vi "Calc Panel Position.vi"(11 "窗格引用":refnum<vi>) -> (3 "Panel Position":T1)   [LabVIEW 2016]
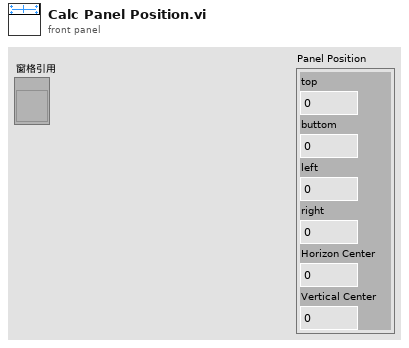
[diagram p1: front panel]
types:
  T1 = cluster{"top":i32, "buttom":i32, "left":i32, "right":i32, "Horizon Center":i32, "Vertical Center":i32}
  T2 = typedef "LVRectTypeDef.ctl" = cluster{"Left":i16, "Top":i16, "Right":i16, "Bottom":i16}
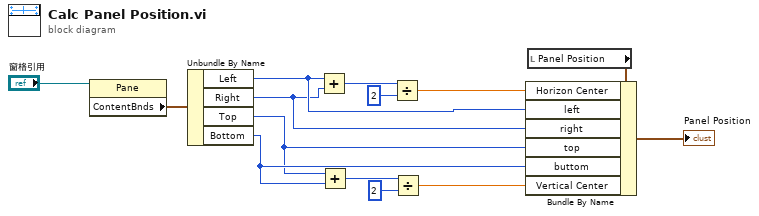
[diagram p0: block diagram]
diagram:
  n1 = property class="Pane"(reference="窗格引用") -> ("ContentBnds"=w10:T2)  [unwired: 1 in, 2 out]
  n2 = Unbundle By Name(w10) -> ("Left"=w7:i16, "Right"=w6:i16, "Top"=w1:i16, "Bottom"=w2:i16)
  n3 = Add(x=w7, y=w6) -> (x+y=w9:i16)
  n4 = Add(x=w1, y=w2) -> (x+y=w5:i16)
  n5 = Divide(x=w9, y=u32 2) -> (x/y=w8:dbl)
  n6 = Divide(x=w5, y=u32 2) -> (x/y=w3:dbl)
  n7 = local read "Panel Position"() -> (w11:T1)
  n8 = Bundle By Name(cluster=w11, "Horizon Center"=w8, "left"=w7, "right"=w6, "top"=w1, "buttom"=w2, "Vertical Center"=w3) -> (→"Panel Position":T1)
